vi "Global_Commands.vi"() -> ()   [LabVIEW 2018]
panel:
  out "J1-B":bool
  out "J1-A":bool
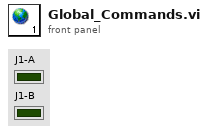
[diagram p1: front panel]
diagram:
